vi "BatchModeStatus.vi"(11 "client handle in":T1) -> (1 "LaserOn?":bool, 2 "batch-mode-pulses-remaining":i32, 3 "client handle out":T1)   [LabVIEW 2020]
uses:
  <vilib>/httpClient/ClientHandle.ctl
  <vilib>/JDP Science/JSONtext/String Subset.vi
  <vilib>/JDP Science/JSONtext/Parsing/Parse Full Path or Item Name.vi
  <vilib>/JDP Science/JSONtext/Next JSON Value.vi
  <vilib>/JDP Science/JSONtext/support/Error Cluster From Code.vi
  <vilib>/JDP Science/JSONtext/Offset/Find Item Locations by Path.vi
  <vilib>/httpClient/LabVIEWHTTPClient.lvlib
  <vilib>/JDP Science/JSONtext/JSONtext.lvlib
panel:
  out "body":string
  out "headers":string
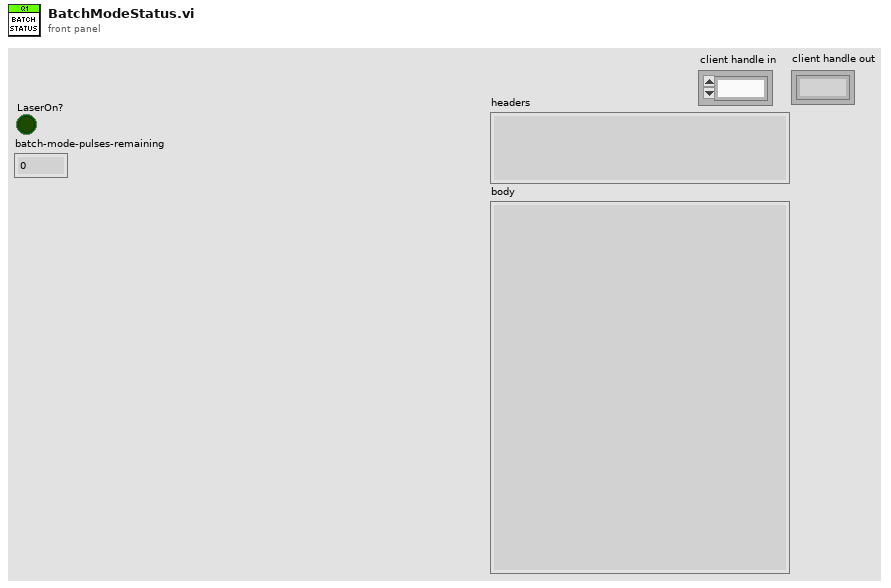
[diagram p1: front panel]
types:
  T1 = typedef "LabVIEWHTTPClient.lvlib/ClientHandle.ctl" = refnum<k1>
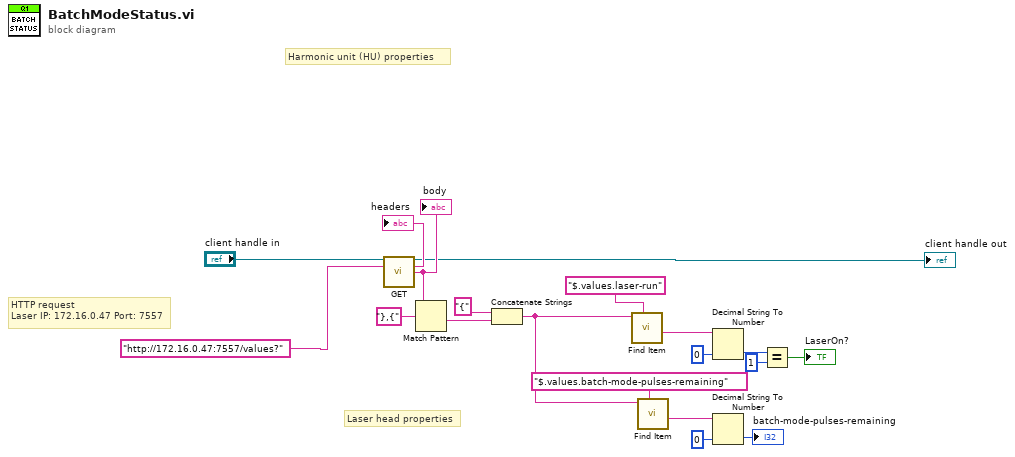
[diagram p0: block diagram]
diagram:
  # "Harmonic unit (HU) properties"
  # "Laser head properties"
  # "HTTP request\nLaser IP: 172.16.0.47 Port: 7557"
  n1 = call <vilib>:"GET.vi"("client handle"="client handle in", "url"="http://172.16.0.47:7557/values?") -> ("client handle out"=→"client handle out":T1, "headers"=→"headers":string, "body"=w3:string)  [unwired: 10 in, 1 out]
  "body" <- w3
  n2 = Match Pattern(string=w3, regular expression="},{") -> (after substring=w14:string)  [unwired: 1 in, 3 out]
  n3 = Concatenate Strings("{" ("string"), w14) -> (w4:string)
  n4 = call <vilib>:"Find Item.vi"("$Path or Item Name"="$.values.laser-run", "JSON"=w4) -> ("<JSON>"=w13:string)  [unwired: 6 in, 3 out]
  n5 = call <vilib>:"Find Item.vi"("$Path or Item Name"="$.values.batch-mode-pulses-remaining", "JSON"=w4) -> ("<JSON>"=w6:string)  [unwired: 6 in, 3 out]
  n6 = Decimal String To Number(string=w13, default (0L)=0 ("default (0 I32)")) -> (number=w11:i32)  [unwired: 1 in, 1 out]
  n7 = Decimal String To Number(string=w6, default (0L)=0 ("default (0 I32)")) -> (number=→"batch-mode-pulses-remaining":i32)  [unwired: 1 in, 1 out]
  n8 = Equal?(x=w11, y=1) -> (x = y?=→"LaserOn?":bool)
